vi "Current_Filepath.vi"(0 "Filename in":path, 1 "Data Type":string="Calibrations") -> (2 "Filename Out":path, 3 "Directory":path)   [LabVIEW 2012]
uses:
  Globals/Meas_global.vi
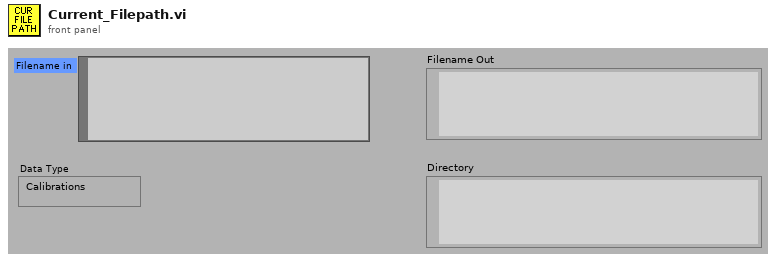
[diagram p1: front panel]
types:
  T1 = typedef "Post_Process.ctl" = enum16{"Take New Data", "Post Process Raw Data File"}
  T2 = typedef "LVDateTimeRec.ctl" = cluster{"fractional second":dbl, "second":i32, "minute":i32, "hour":i32, "day of month":i32, "month":i32, "year":i32, "day of week":i32, "day of year":i32, "DST":i32}
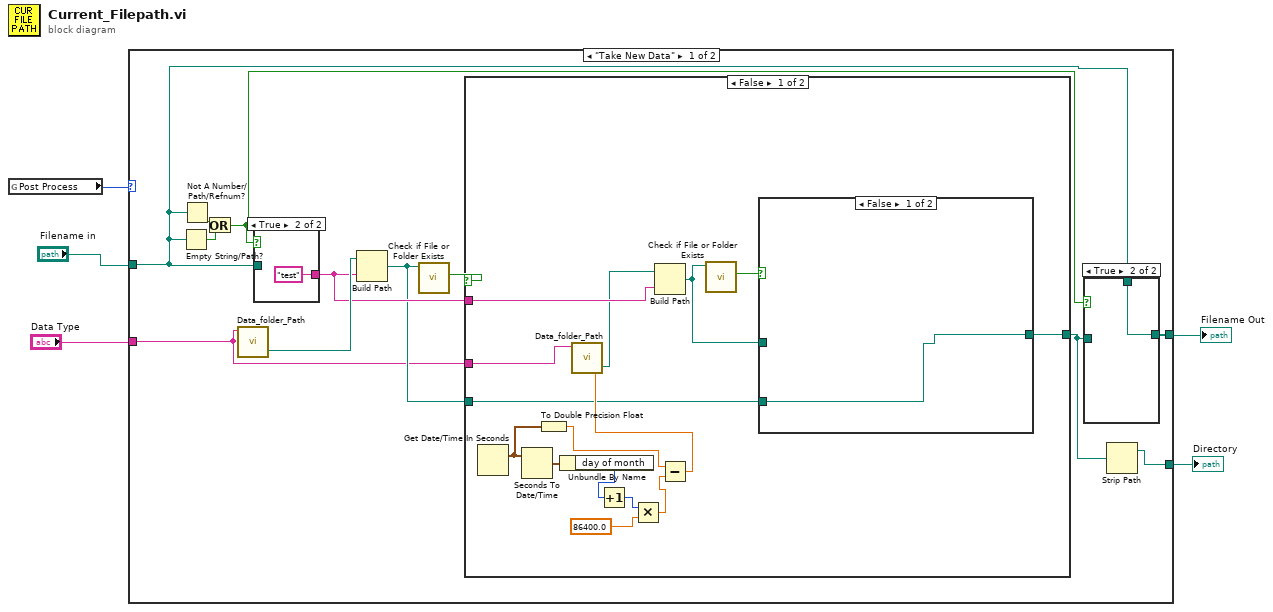
[diagram p0: block diagram]
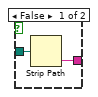
[diagram p3: hidden frame]
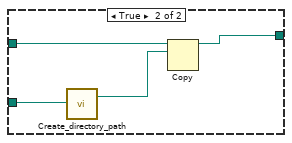
[diagram p4: hidden frame]
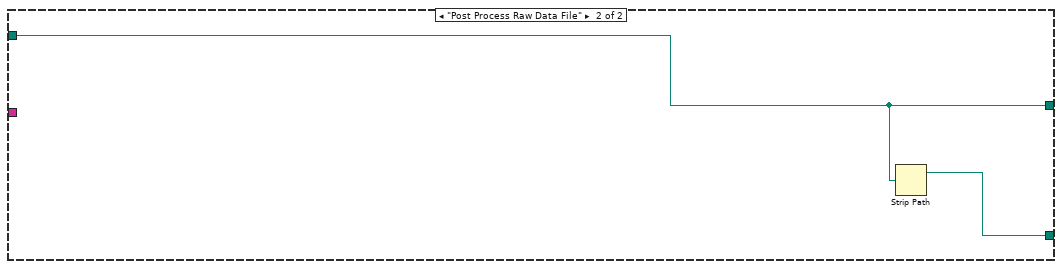
[diagram p6: hidden frame]
diagram:
  n1 = global read "Meas_global.vi" "Post Process"() -> (w2:T1)
  n2 = case shown="\"Take New Data\"" w2 {
    tunnel: "Filename in" -> [w6 w45]
    tunnel: "Data Type" -> [w13 _]
    tunnel: [w9 w45] -> w3
    tunnel: [w7 w44] -> w1
    frame "Take New Data" {
      n3 = Empty String/Path?(string/path=w6) -> (empty?=w11:bool)
      n4 = Not A Number/Path/Refnum?(number/path/refnum=w6) -> (NaN/Path/Refnum?=w12:bool)
      n5 = Or(x=w12, y=w11) -> (x .or. y?=w10:bool)
      n6 = call "Data_folder_Path.vi"("Data Type"=w13) -> ("Data Folder"=w17:path)  [unwired: 4 in]
      n7 = case shown="True" w10 {
        tunnel: [w21 "test" ("name")] -> w15
        tunnel: w6 -> [w20 _]
        frame False {
          n8 = Strip Path(path=w20) -> (name=w21:string)  [unwired: 1 out]
        }
        frame True {
        }
      }
      n9 = Build Path(base path=w17, name or relative path=w15) -> (appended path=w14:path)
      n10 = call <vilib>:"Check if File or Folder Exists.vi"("path"=w14) -> ("file or folder exists?"=w16:bool)  [unwired: 1 in, 9 out]
      n11 = case shown="False" w16 {
        tunnel: w13 -> [w30 _]
        tunnel: w15 -> [w36 _]
        tunnel: w14 -> [w33 w43]
        tunnel: [w31 w43] -> w8
        frame False {
          n12 = Get Date/Time In Seconds() -> (seconds since 1Jan1904=w24:timestamp)
          n13 = Seconds To Date/Time(time stamp (now)=w24) -> (date time rec=w29:T2)  [unwired: 1 in]
          n14 = To Double Precision Float(number=w24) -> (double precision float=w23:dbl)
          n15 = Unbundle By Name(w29) -> ("day of month"=w28:i32)
          n16 = Increment(x=w28) -> (x+1=w27:i32)
          n17 = Multiply(x=w27, y=86400.0) -> (x*y=w25:dbl)
          n18 = Subtract(x=w23, y=w25) -> (x-y=w37:dbl)
          n19 = call "Data_folder_Path.vi"("seconds"=w37, "Data Type"=w30) -> ("Data Folder"=w34:path)  [unwired: 3 in]
          n20 = Build Path(base path=w34, name or relative path=w36) -> (appended path=w32:path)
          n21 = call <vilib>:"Check if File or Folder Exists.vi"("path"=w32) -> ("file or folder exists?"=w35:bool)  [unwired: 1 in, 9 out]
          n22 = case shown="False" w35 {
            tunnel: w32 -> [_ w42]
            tunnel: w33 -> [w38 w40]
            tunnel: [w38 w41] -> w31
            frame False {
            }
            frame True {
              n23 = call "Create_directory_path.vi"("Path name"=w40) -> ("Path name Out"=w39:path)  [unwired: 1 in, 1 out]
              n24 = Copy(10:w39, 11:w42) -> (3:w41:path)  [unwired: 3 in, 2 out]
            }
          }
        }
        frame True {
        }
      }
      n25 = case shown="True" w10 {
        tunnel: w8 -> [w18 _]
        tunnel: [w18 w19] -> w9
        tunnel: w6 -> [_ w19]
        frame False {
        }
        frame True {
        }
      }
      n26 = Strip Path(path=w8) -> (stripped path=w7:path)  [unwired: 1 out]
    }
    frame "Post Process Raw Data File" {
      n27 = Strip Path(path=w45) -> (stripped path=w44:path)  [unwired: 1 out]
    }
  }
  "Filename Out" <- w3
  "Directory" <- w1
